vi "Write Asymmetric.vi"(8 "error in (no error)":errorcluster, 10 "Asymmetric":bool, 11 "Gate in":refnum<class "Gate.lvclass">) -> (0 "error out":errorcluster, 3 "Gate out":refnum<class "Gate.lvclass">)   [LabVIEW 2020, in "Gate.lvclass"]
uses:
  Gate.lvclass
  Gate.lvclass/Gate.ctl
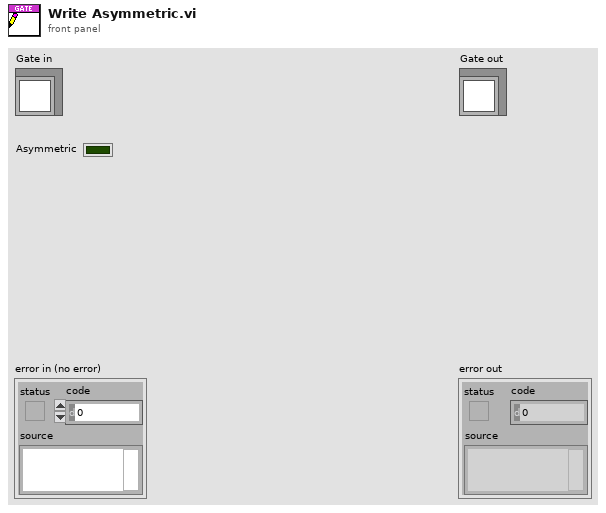
[diagram p1: front panel]
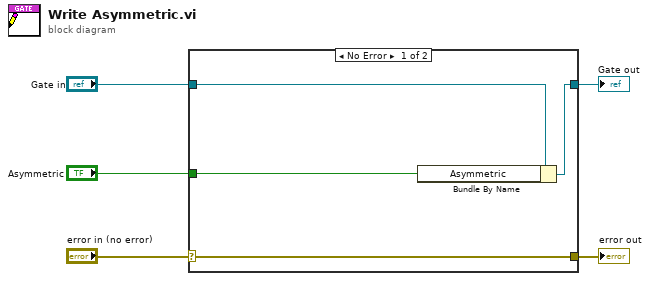
[diagram p0: block diagram]
diagram:
  n1 = case shown="No Error" "error in (no error)" {
    selector: "error in (no error)" -> [w9 w10]
    tunnel: [w9 w10] -> w4
    tunnel: [w7 w11] -> w2
    tunnel: "Gate in" -> [w8 w11]
    tunnel: "Asymmetric" -> [w6 _]
    frame No Error {
      n2 = Bundle By Name(cluster=w8, "Asymmetric"=w6) -> (w7:refnum<class "Gate.lvclass">)
    }
    frame Error {
    }
  }
  "error out" <- w4
  "Gate out" <- w2
